vi "GetKeyValue.vi"(6 "default value":string, 9 "key":string, 10 "key value pairs":T1[](array[typedef])) -> (1 "value":string, 2 "key value pairs out":T1[](array[typedef]), 5 "found":bool)   [LabVIEW 2017, in "PropertyHelpers.lvlib"]
doc: "Returns the string value of a particular key in an array of key-value pairs. Use this VI to get properties from the contents of configuration JSON files that the Global Configuration VIs return."
uses:
  <vilib>/addons/InsightCM/Utilities/PropertyHelpers/PropertyHelpers.lvlib
  <vilib>/addons/InsightCM/MessageBus/Base/controls/KeyValuePair.ctl
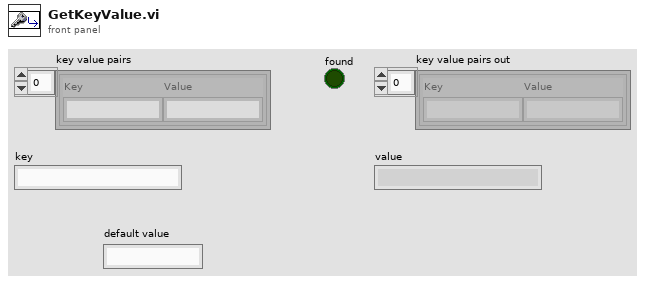
[diagram p1: front panel]
types:
  T1 = typedef "KeyValuePair.ctl" = cluster{"Key":string, "Value":string}
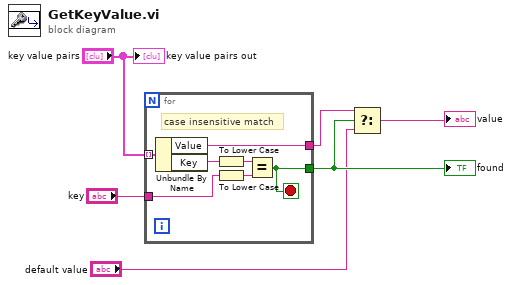
[diagram p0: block diagram]
diagram:
  n1 = for {
    tunnel: "key value pairs" -> [w13] mode=indexing
    tunnel: "key" -> [w7]
    tunnel: [w12] -> w3
    tunnel: [w11] -> w4
    stop <- w12 stop-if-true
    # "case insensitive match"
    n2 = Unbundle By Name(w13) -> ("Value"=w11:string, "Key"=w10:string)
    n3 = To Lower Case(string=w10) -> (all lower case string=w9:string)
    n4 = To Lower Case(string=w7) -> (all lower case string=w8:string)
    n5 = Equal?(x=w9, y=w8) -> (x = y?=w12:bool)
  }
  "found" <- w3
  n6 = Select(t=w4, s=w3, f="default value") -> (s? t:f=→"value":string)
  "key value pairs out" <- "key value pairs"
